vi "moveWaitUntilDone_checkPressureNotPos.vi"(4 "Accuracy":dbl, 5 "ArduinoHandle":T1={"VISA resource"="", "Board Type"=enum."Uno", "Connection Type"=enum."USB / Serial", "Bytes Per Packet (15)"=15}, 6 "Transducer (psi)":dbl(ring)=1.0 items=["+/- .18 psi"=1.0, "+/- .36 psi"=2.0, "+/- 1.08 psi"=3.0], 7 "Position (mm)":dbl(slide)=1.0 min=0.0 max=100.0 step=0.1 scale=0.0..100.0 scale format="%.2f", 8 "Pressure (psi)":dbl, 9 "maxLength":dbl, 10 "PressureOffset":dbl, 11 "WRITE_HANDLE":u32 format="%04x") -> (1 "moveDone?":bool, 3 "regSetting":u16)   [LabVIEW 2011]
uses:
  <vilib>/LabVIEW Interface for Arduino/Type Defs/Arduino Resource.ctl
  <vilib>/LabVIEW Interface for Arduino/Type Defs/Board Type.ctl
  <vilib>/LabVIEW Interface for Arduino/LabVIEW Interface for Arduino.lvlib
panel:
  in  "stop":bool
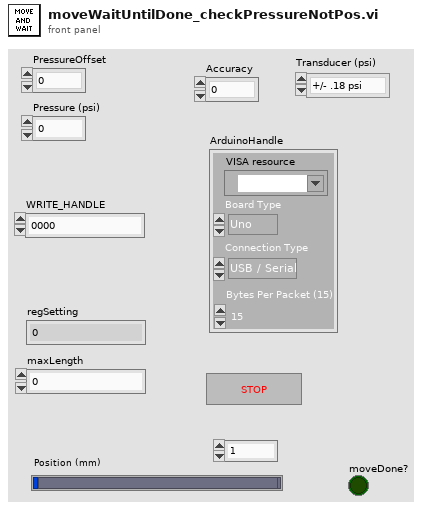
[diagram p1: front panel]
types:
  T1 = typedef "LabVIEW Interface for Arduino.lvlib/Arduino Resource.ctl" = cluster{"VISA resource":refnum<visa-resource-name>, "Board Type":T2, "Connection Type":enum8{"USB / Serial"}, "Bytes Per Packet (15)":u8}
  T2 = typedef "LabVIEW Interface for Arduino.lvlib/Board Type.ctl" = enum16{"Uno", "Dimuelanove w/Atmega 328", "Mega 2560"}
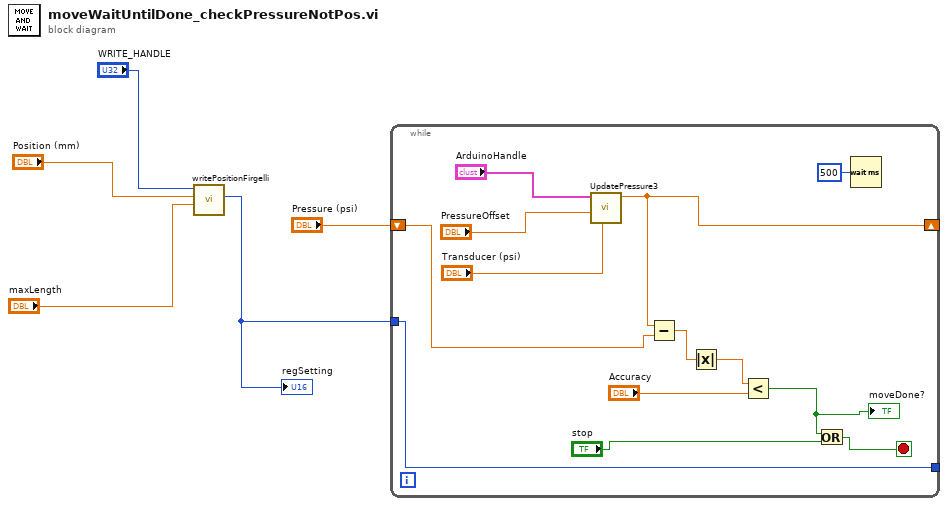
[diagram p0: block diagram]
diagram:
  n1 = call "writePositionFirgelli.vi"("lengthMax"="maxLength", "Position (mm)"="Position (mm)", "handleIn"="WRITE_HANDLE") -> ("regSetting"=w1:u16)  [unwired: 1 in, 7 out]
  "regSetting" <- w1
  n2 = while {
    shift-right: [w16] -> _
    shift-left: "Pressure (psi)" -> [w17]
    tunnel: w1 -> [w6]
    tunnel: [w6] -> _
    stop <- w13 stop-if-true
    n3 = call "UpdatePressure3.vi"("Transducer (psi)"="Transducer (psi)", "PressureOffset"="PressureOffset", "ArduinoHandle"="ArduinoHandle") -> ("Pressure (psi)"=w16:dbl)  [unwired: 7 in, 1 out]
    n4 = Subtract(x=w16, y=w17) -> (x-y=w18:dbl)
    n5 = Absolute Value(x=w18) -> (abs(x)=w15:dbl)
    n6 = Less?(x=w15, y="Accuracy") -> (x < y?=w12:bool)
    "moveDone?" <- w12
    n7 = Or(x=w12, y="stop") -> (x .or. y?=w13:bool)
    n8 = Wait (ms)(milliseconds to wait=u32 500) -> ()  [unwired: 1 out]
  }
